vi "Fetch Waveforms.vi"(8 "error in":errorcluster, 11 "object in":refnum<class "Scope PXI CFG.lvclass">) -> (0 "error out":errorcluster, 2 "Last Waveforms":map{u8, waveform(dbl)}(c390), 3 "object out":refnum<class "Scope PXI CFG.lvclass">)   [LabVIEW 2023, in "Scope.lvlib" / "Scope PXI.lvlib" / "Scope PXI CFG.lvclass"]
uses:
  Scope PXI CFG.lvclass
  D:/git/HAL/Configuration Base/Configuration Base.lvclass
  Scope PXI CFG.lvclass/Scope PXI CFG.ctl
  Configuration Base/Configuration Base.lvclass/Configuration Base.ctl
  <instrlib>/niScope/Controls/niScope timestamp type.ctl
  d9bd0854-c9e2-4517-b292-7db69c37fda0.vi
  8d36052f-398f-4416-96a9-5ca09e3acc97.vi
  ce682fe7-8147-45a0-826f-6225c648e612.vi
  02167e95-eb1b-459e-9628-7c497ad36d0b.vi
  <vilib>/JDP Science/JSONtext/Find Item.vi
  <vilib>/JDP Science/JSONtext/Next JSON Value.vi
  <vilib>/JDP Science/JSONtext/String Subset.vi
  <vilib>/JDP Science/JSONtext/Parsing/Advance past next JSON Value (inlined COPY).vi
  <vilib>/JDP Science/JSONtext/Parsing/Advance past whitespace.vi
  <vilib>/JDP Science/JSONtext/Parsing/Advance past String.vi
  <vilib>/JDP Science/JSONtext/Parsing/Advance past Number.vi
  <vilib>/JDP Science/JSONtext/Parsing/Advance past Line Ending.vi
  <vilib>/JDP Science/JSONtext/Parsing/Parse Full Path or Item Name.vi
  <vilib>/JDP Science/JSONtext/Parsing/Advance past Array.vi
  <vilib>/JDP Science/JSONtext/Parsing/Advance past Object.vi
  <vilib>/JDP Science/JSONtext/support/Error Cluster From Code.vi
  <vilib>/JDP Science/JSONtext/Offset/Find Item Locations by Path.vi
  <vilib>/JDP Science/JSONtext/JSON text to Variant.vi
  <vilib>/Utility/error.llb/Error Cluster From Error Code.vi
  <instrlib>/niScope/Acquire/Fetch/niScope Fetch WDT.vi
  <vilib>/JDP Science/JSONtext/LVClass Serializer/JSONtext LVClass Serializer.lvclass
  <vilib>/ErrorRing/Error Ring.xnode
  Configuration Base/Configuration Base.lvclass
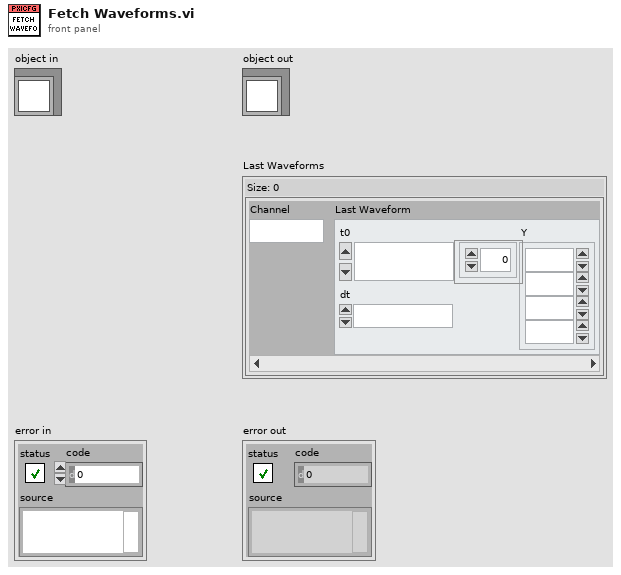
[diagram p1: front panel]
types:
  T1 = typedef "niScope timestamp type.ctl" = i32
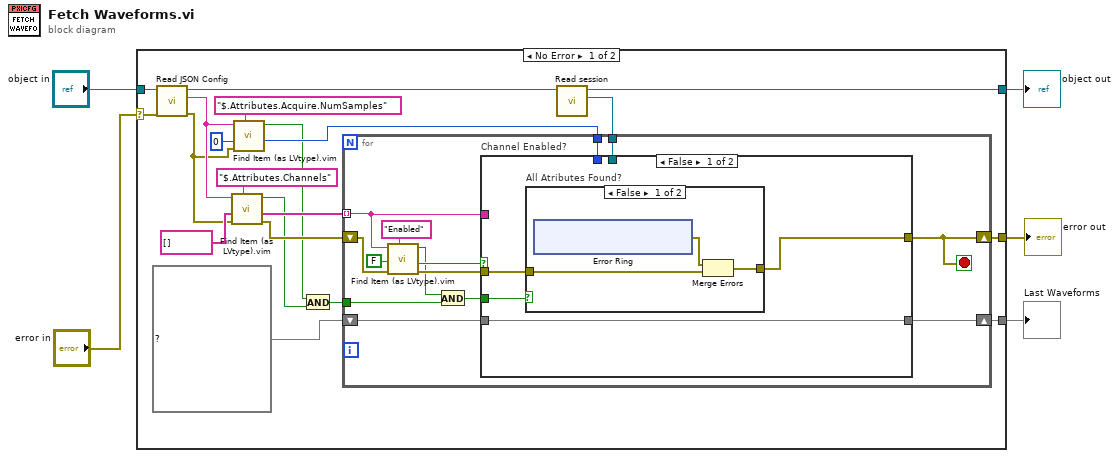
[diagram p0: block diagram]
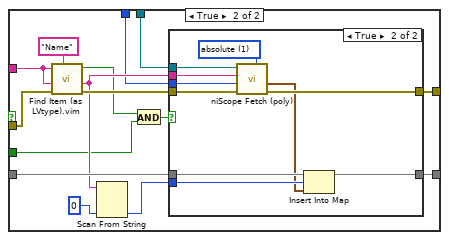
[diagram p3: hidden frame]
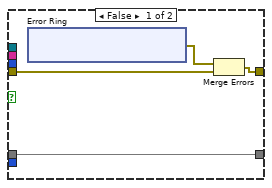
[diagram p4: hidden frame]
diagram:
  n1 = case shown="No Error" "error in" {
    selector: "error in" -> [w14 w88]
    tunnel: [w25 w87] -> w5
    tunnel: "object in" -> [w24 w87]
    tunnel: [w16 _] -> w3
    tunnel: [w15 w88] -> w2
    frame No Error {
      n2 = call "Read JSON Config.vi"("error in"=w14, "object in"=w24) -> ("error out"=w11:errorcluster, "<JSON>Config"=w13:string, "object out"=w23:refnum<class "Scope PXI CFG.lvclass">)  [unwired: 7 in]
      n3 = call "Find Item (as LVtype).vim"("$Path or Item Name"="$.Attributes.Channels", "error in (no error)"=w11, "Data Type and Default Value"=string[] [], "JSON"=w13) -> ("error out"=w19:errorcluster, "Data"=w20:string[], "Found"=w7:bool)  [unwired: 4 in, 1 out]
      n4 = call "Find Item (as LVtype).vim"("$Path or Item Name"="$.Attributes.Acquire.NumSamples", "error in (no error)"=w11, "Data Type and Default Value"=0, "JSON"=w13) -> ("Data"=w9:i32, "Found"=w8:bool)  [unwired: 4 in, 2 out]
      n5 = And(x=w8, y=w7) -> (x .and. y?=w6:bool)
      n6 = call "Read session.vi"("Scope PXI CFG in"=w23) -> ("session"=w18:refnum<k15>, "Scope PXI CFG out"=w25:refnum<class "Scope PXI CFG.lvclass">)  [unwired: 8 in, 1 out]
      n7 = for {
        tunnel: w20 -> [w34] mode=indexing
        tunnel: w18 -> [w33]
        shift-right: [w26] -> w15
        shift-left: w19 -> [w39]
        shift-right: [w31] -> w16
        shift-left: map{u8, waveform(dbl)} {} ("Last Waveforms") -> [w32]
        tunnel: w9 -> [w30]
        tunnel: w6 -> [w27]
        stop <- w26 stop-if-true
        n8 = call "Find Item (as LVtype).vim"("$Path or Item Name"="Enabled", "error in (no error)"=w39, "Data Type and Default Value"=FALSE, "JSON"=w34) -> ("error out"=w36:errorcluster, "Data"=w35:bool, "Found"=w29:bool)  [unwired: 4 in, 1 out]
        n9 = And(x=w29, y=w27) -> (x .and. y?=w28:bool)
        n10 = case "Channel Enabled?" shown="False" w35 {
          tunnel: w36 -> [w41 w67]
          tunnel: w34 -> [_ w60]
          tunnel: w33 -> [_ w65]
          tunnel: [w40 w63] -> w26
          tunnel: w32 -> [w43 w62]
          tunnel: [w43 w61] -> w31
          tunnel: w30 -> [_ w56]
          tunnel: w28 -> [w42 w53]
          frame False {
            n11 = case "All Atributes Found?" shown="False" w42 {
              tunnel: w41 -> [w46 w52]
              tunnel: [w44 w52] -> w40
              frame False {
                n12 = xnode "Error Ring"() -> ("error out"=w45:errorcluster)
                n13 = Merge Errors(w45, w46) -> (w44:errorcluster)
              }
              frame True {
              }
            }
          }
          frame True {
            n14 = call "Find Item (as LVtype).vim"("$Path or Item Name"="Name", "error in (no error)"=w67, "Data Type and Default Value"=w60, "JSON"=w60) -> ("error out"=w64:errorcluster, "Data"=w59:string, "Found"=w54:bool)  [unwired: 4 in, 1 out]
            n15 = Scan From String(input string=w59, default 1=u8 0 ("key")) -> (output 1=w57:u8)  [unwired: 3 in, 3 out]
            n16 = And(x=w54, y=w53) -> (x .and. y?=w55:bool)
            n17 = case shown="True" w55 {
              tunnel: w65 -> [_ w86]
              tunnel: w64 -> [w71 w85]
              tunnel: [w69 w84] -> w63
              tunnel: w62 -> [w70 w83]
              tunnel: [w70 w82] -> w61
              tunnel: w59 -> [_ w81]
              tunnel: w57 -> [_ w80]
              tunnel: w56 -> [_ w77]
              frame False {
                n18 = xnode "Error Ring"() -> ("error out"=w68:errorcluster)
                n19 = Merge Errors(w68, w71) -> (w69:errorcluster)
              }
              frame True {
                w78 = T1 1 items=["relative", "absolute"] ("timestamp Type")
                n20 = call-poly <instrlib>:"niScope Fetch (poly).vi"("timestamp Type"=w78, "error in"=w85, "numSamples"=w77, "channels"=w81, "instrument handle"=w86) -> ("error out"=w84:errorcluster, "wfm"=w79:waveform(dbl))  [unwired: 3 in, 2 out]
                n21 = Insert Into Map(map in=w83, key=w80, value=w79) -> (map out=w82:map{u8, waveform(dbl)})  [unwired: 2 out]
              }
            }
          }
        }
      }
    }
    frame Error {
    }
  }
  "error out" <- w2
  "object out" <- w5
  "Last Waveforms" <- w3
